vi "ADC_BulkPoll.vi"(7 "DeviceIndex":u32, 8 "error in (no error)":errorcluster) -> (0 "error out":errorcluster, 3 "BytesLeft":u32)   [LabVIEW 2012]
doc: "Use ADC_BulkPoll() to query the status of this background operation.\nunsigned long ADC_BulkPoll(\nunsigned long DeviceIndex - number from 0-31 indicating from which device you wish to query\nA/D status\nunsigned long *BytesLeft - a pointer to a variable which will be set to the number of bytes of\nA/D data remaining to be taken\n)\nNote that any data that has been taken is available in the buffer, starting from the beginning. For\nexample, if ADC_BulkAcquire() was called to take 1024 MB of data, and ADC_BulkPoll()\nindicates 768 MB remains to be taken, the first 256 MB of data is available."
uses:
  Windows/System32/AIOUSB.dll
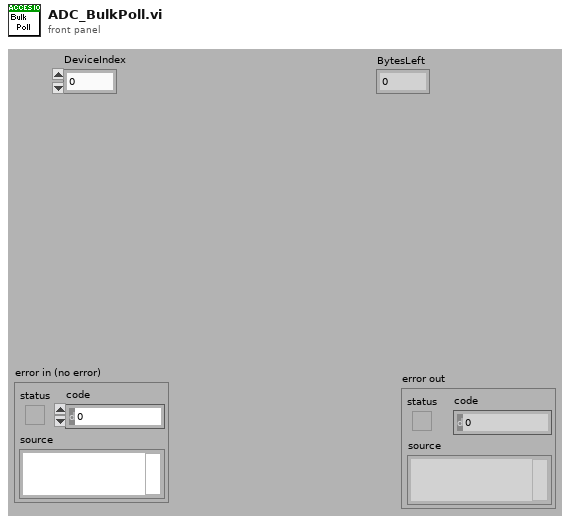
[diagram p1: front panel]
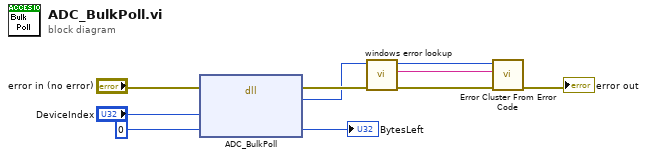
[diagram p0: block diagram]
diagram:
  n1 = dll-call lib="C:/Windows/System32/AIOUSB.dll" fn="ADC_BulkPoll"(error in="error in (no error)", "DeviceIndex"="DeviceIndex", "BytesLeft"=u32 0 ("BufSize")) -> (error out=w4:errorcluster, "return type"=w1:u32, "BytesLeft"=→"BytesLeft":u32)  [unwired: 3 in, 1 out]
  n2 = call "windows error lookup.vi"("error in (no error)"=w4, "Error Code"=w1) -> ("error out"=w3:errorcluster, "error message (\"\")"=w2:string)  [unwired: 8 in]
  n3 = call <vilib>:"Error Cluster From Error Code.vi"("error in (no error)"=w3, "error message (\"\")"=w2, "error code (0)"=w1) -> ("error out"=→"error out":errorcluster)  [unwired: 6 in]
